vi "Init.vi"() -> (6 "ExecAnchor out":refnum<class "ExecAnchor.lvclass">)   [LabVIEW 2020, in "ExecAnchor.lvclass"]
uses:
  ExecAnchor.lvclass
  ExecAnchor.lvclass/ExecAnchor.ctl
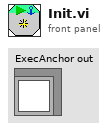
[diagram p1: front panel]
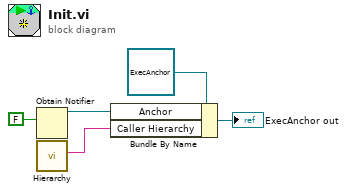
[diagram p0: block diagram]
diagram:
  n1 = Obtain Notifier(notification data type=FALSE) -> (notifier out=w3:refnum<notifier>)  [unwired: 3 in, 2 out]
  n2 = call "Hierarchy.vi"() -> ("Hierarchy"=w1:string)  [unwired: 11 in]
  n3 = Bundle By Name(cluster=refnum<class "ExecAnchor.lvclass"> refnum ("ExecAnchor in"), "Anchor"=w3, "Caller Hierarchy"=w1) -> (→"ExecAnchor out":refnum<class "ExecAnchor.lvclass">)
